vi "(Sub) Elapsed Time.vi"(8 "error in (no error)":errorcluster caption="에러 입력(에러 없음)", 11 "In ms":u32) -> (0 "error out":errorcluster caption="에러 출력", 1 "S":string, 2 "M":string, 3 "H":string)   [LabVIEW 2017]
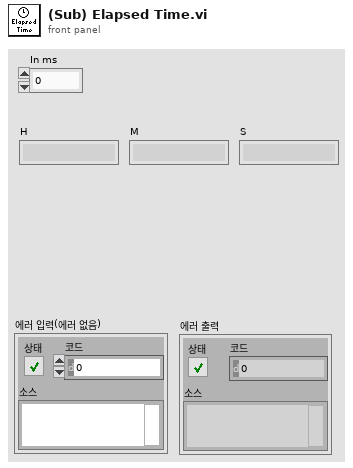
[diagram p1: front panel]
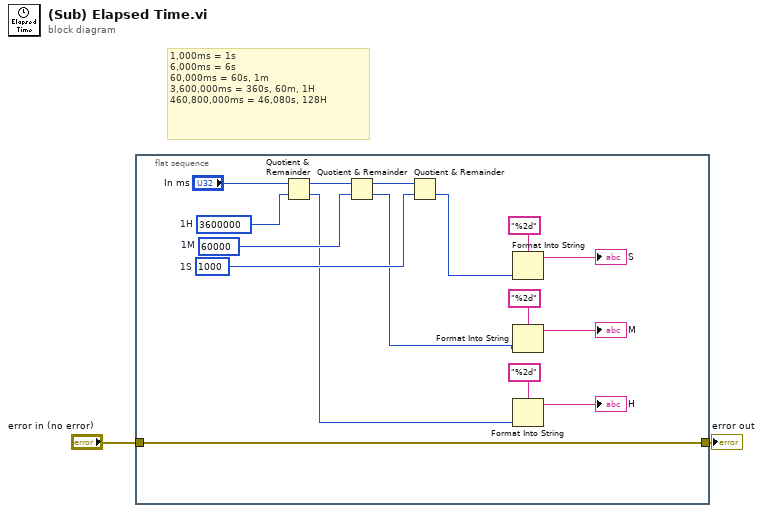
[diagram p0: block diagram]
diagram:
  # "1,000ms = 1s\n6,000ms = 6s\n60,000ms = 60s, 1m\n3,600,000ms = 360s, 60m, 1H\n460,800,000ms = 46,080s, 128H"
  n1 = flat-sequence {
    tunnel: "error in (no error)" -> [w12]
    tunnel: [w12] -> w1
    frame #0 {
      w14 = u32 1000  # 1S
      w16 = u32 60000  # 1M
      w18 = u32 3600000  # 1H
      n2 = Quotient & Remainder(x="In ms", y=w18) -> (x-y*floor(x/y)=w17:u32, floor(x/y)=w5:u32)
      n3 = Quotient & Remainder(x=w17, y=w16) -> (x-y*floor(x/y)=w15:u32, floor(x/y)=w8:u32)
      n4 = Quotient & Remainder(x=w15, y=w14) -> (floor(x/y)=w11:u32)  [unwired: 1 out]
      n5 = Format Into String(format string="%2d" ("포맷 문자열"), w11) -> (resulting string=→"S":string)  [unwired: 2 in, 1 out]
      n6 = Format Into String(format string="%2d" ("포맷 문자열"), w8) -> (resulting string=→"M":string)  [unwired: 2 in, 1 out]
      n7 = Format Into String(format string="%2d" ("포맷 문자열"), w5) -> (resulting string=→"H":string)  [unwired: 2 in, 1 out]
    }
  }
  "error out" <- w1
